vi "Get_LV_Printing_Color_Setting.vi"(0 "error in (no error)":errorcluster) -> (1 "Color?":T1 items=["Unchanged", "Color/grayscale", "Monochrome"], 2 "error out":errorcluster)   [LabVIEW 2020, in "NI_ReportGenerationCore.lvlib"]
uses:
  <vilib>/Utility/NIReport.llb/NI_ReportGenerationCore.lvlib
  <vilib>/printing/EasyPrintingControls.llb/color_or_monochrome.ctl
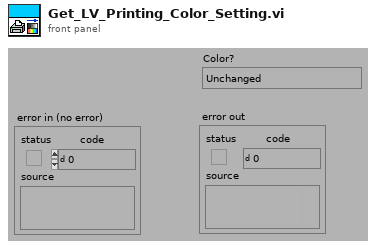
[diagram p1: front panel]
types:
  T1 = typedef "NI_ReportGenerationCore.lvlib/color_or_monochrome.ctl" = u16
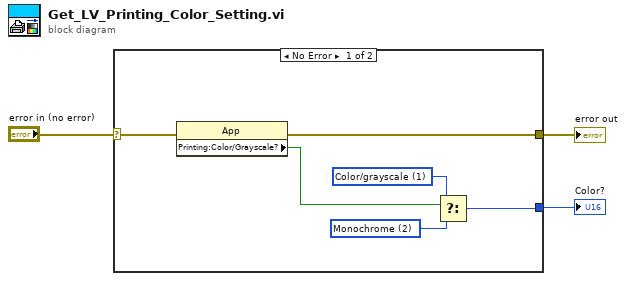
[diagram p0: block diagram]
diagram:
  n1 = case shown="No Error" "error in (no error)" {
    selector: "error in (no error)" -> [w6 w10]
    tunnel: [w5 w10] -> w2
    tunnel: [w4 _] -> w1
    frame No Error {
      w8 = T1 1 items=["Unchanged", "Color/grayscale", "Monochrome"] ("color or monochrome")
      w7 = T1 2 items=["Unchanged", "Color/grayscale", "Monochrome"] ("color or monochrome")
      n2 = property class="App"(error in=w6) -> (error out=w5:errorcluster, "Printing:Color/Grayscale?"=w9:bool)  [unwired: 1 in, 1 out]
      n3 = Select(t=w8, s=w9, f=w7) -> (s? t:f=w4:T1)
    }
    frame Error {
    }
  }
  "error out" <- w2
  "Color?" <- w1
